vi "escreve_analogico.vi"() -> ()   [LabVIEW 2020]
uses:
  <vilib>/DAQmx/write.llb/DAQmx Write (Analog DBL 1Chan 1Samp).vi
  <vilib>/DAQmx/create/channels.llb/DAQmx Create Channel (AO-Voltage-Basic).vi
  <vilib>/DAQmx/miscellaneous.llb/DAQmx Fill In Error Info.vi
panel:
  in  "physical channels":tag
  out "error out":errorcluster
  out "task out 2":refnum<k21>
  in  "task out":refnum<k21>
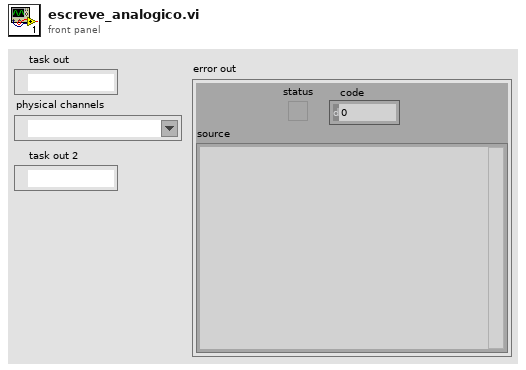
[diagram p1: front panel]
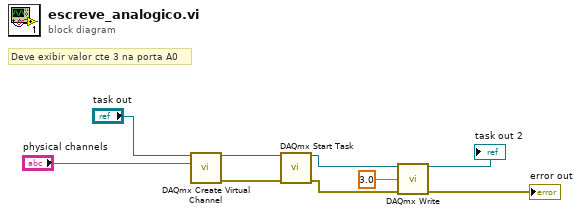
[diagram p0: block diagram]
diagram:
  # "Deve exibir valor cte 3 na porta A0"
  n1 = call-poly <vilib>:"DAQmx Create Virtual Channel.vi"("task in"="task out", "physical channels"="physical channels") -> ("task out"=w9:refnum<k21>, "error out"=w5:errorcluster)  [unwired: 12 in]
  n2 = call <vilib>:"DAQmx Start Task.vi"("task/channels in"=w9, "error in"=w5) -> ("task out"=w8:refnum<k21>, "error out"=w4:errorcluster)  [unwired: 12 in]
  n3 = call-poly <vilib>:"DAQmx Write.vi"("task/channels in"=w8, "data"=3.0, "error in"=w4) -> ("task out"=→"task out 2":refnum<k21>, "error out"=→"error out":errorcluster)  [unwired: 10 in, 1 out]
